vi "(Loop) HVPS_1.vi"   [LabVIEW 2017]
uses:
  Controls/(Ctrl) State_HVPS CMD.ctl
  Variables/(Var) System.vi
  Variables/(Var) Get_HVPS_1.vi
types:
  T1 = typedef "(Ctrl) State_HVPS CMD.ctl" = enum16{"Open", "Rx : V", "Rx : mA", "Rx : State", "Rx : ADC", "Tx : Set V", "Tx : Set mA", "Tx : ON", "Tx : OFF", "Close"}
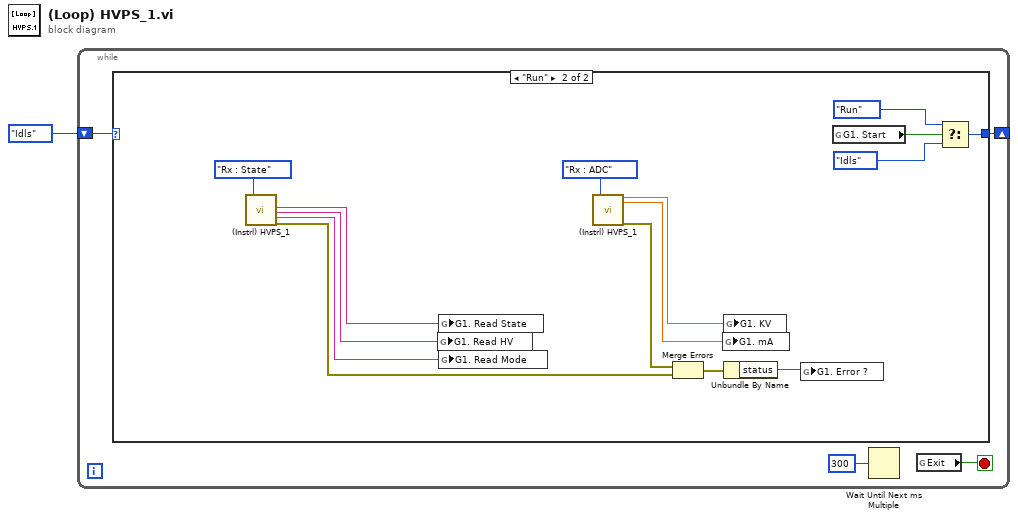
[diagram p0: block diagram]
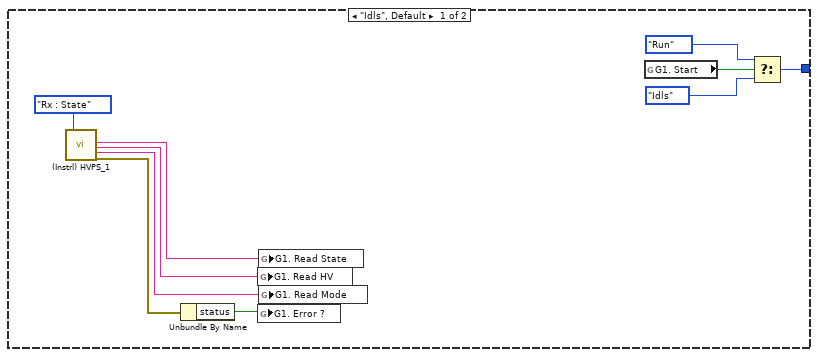
[diagram p2: hidden frame]
diagram:
  n1 = while {
    shift-right: [w2] -> _
    shift-left: enum16{"Init", "Idls", "Run", "Stop", "Close"}."Idls" -> [w4]
    stop <- w5 stop-if-true
    n2 = case shown="\"Run\"" w4 {
      tunnel: [w6 w22] -> w2
      frame "Idls", Default {
        n3 = call "(Instrl) HVPS_1.vi"("CMD"=(Ctrl)_State_HVPS_CMD."Rx : State" ("State")) -> ("System State"=w12:string, "HV State"=w11:string, "Operation Mode"=w10:string, "error out"=w14:errorcluster)  [unwired: 13 in, 2 out]
        n4 = Unbundle By Name(w14) -> ("status"=w13:bool)
        n5 = global write "(Var) Get_HVPS_1.vi" "G1. Read HV"(w11) -> ()
        n6 = global write "(Var) Get_HVPS_1.vi" "G1. Error ?"(w13) -> ()
        n7 = global write "(Var) Get_HVPS_1.vi" "G1. Read State"(w12) -> ()
        n8 = global write "(Var) Get_HVPS_1.vi" "G1. Read Mode"(w10) -> ()
        n9 = global read "(Var) Get_HVPS_1.vi" "G1. Start"() -> (w9:bool)
        n10 = Select(t=enum16{"Init", "Idls", "Run", "Stop", "Close"}."Run", s=w9, f=enum16{"Init", "Idls", "Run", "Stop", "Close"}."Idls") -> (s? t:f=w6:enum16{"Init", "Idls", "Run", "Stop", "Close"})
      }
      frame "Run" {
        n11 = call "(Instrl) HVPS_1.vi"("CMD"=(Ctrl)_State_HVPS_CMD."Rx : State" ("State")) -> ("System State"=w28:string, "HV State"=w27:string, "Operation Mode"=w26:string, "error out"=w16:errorcluster)  [unwired: 13 in, 2 out]
        n12 = global write "(Var) Get_HVPS_1.vi" "G1. Read HV"(w27) -> ()
        n13 = global write "(Var) Get_HVPS_1.vi" "G1. Read State"(w28) -> ()
        n14 = global write "(Var) Get_HVPS_1.vi" "G1. Read Mode"(w26) -> ()
        n15 = call "(Instrl) HVPS_1.vi"("CMD"=(Ctrl)_State_HVPS_CMD."Rx : ADC" ("State")) -> ("Get V"=w20:dbl, "Get mA"=w19:dbl, "error out"=w17:errorcluster)  [unwired: 13 in, 3 out]
        n16 = Merge Errors(w17, w16) -> (w18:errorcluster)
        n17 = global write "(Var) Get_HVPS_1.vi" "G1. mA"(w19) -> ()
        n18 = global write "(Var) Get_HVPS_1.vi" "G1. KV"(w20) -> ()
        n19 = Unbundle By Name(w18) -> ("status"=w29:bool)
        n20 = global write "(Var) Get_HVPS_1.vi" "G1. Error ?"(w29) -> ()
        n21 = global read "(Var) Get_HVPS_1.vi" "G1. Start"() -> (w25:bool)
        n22 = Select(t=enum16{"Init", "Idls", "Run", "Stop", "Close"}."Run", s=w25, f=enum16{"Init", "Idls", "Run", "Stop", "Close"}."Idls") -> (s? t:f=w22:enum16{"Init", "Idls", "Run", "Stop", "Close"})
      }
    }
    n23 = Wait Until Next ms Multiple(millisecond multiple=u32 300 ("대기 시간 (ms)")) -> ()  [unwired: 1 out]
    n24 = global read "(Var) System.vi" "Exit"() -> (w5:bool)
  }
